vi "Set Subpanel Status.vi"(0 "GUI Container in":refnum<class "GUI Container.lvclass">, 5 "Subpanel":string, 9 "Subpanel Status":T1, 11 "error in (no error)":errorcluster) -> (4 "GUI Container out":refnum<class "GUI Container.lvclass">, 8 "Status Added":bool, 15 "error out":errorcluster)   [LabVIEW 2023, in "GUI Views.lvlib" / "GUI Container.lvclass"]
uses:
  GUI Container.lvclass
  typedefs/Subpanel Status.ctl
  GUI Container.lvclass/GUI Container.ctl
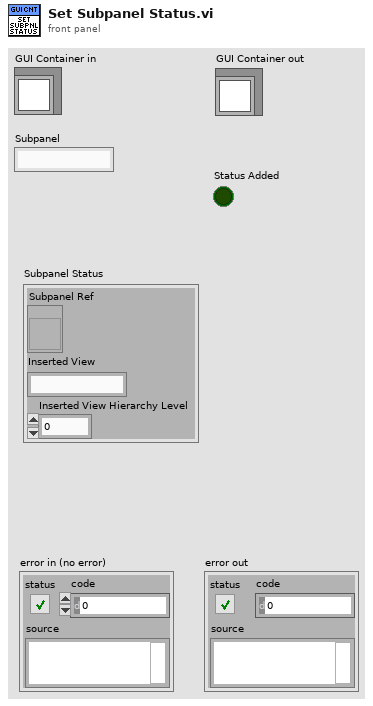
[diagram p1: front panel]
types:
  T1 = typedef "GUI Views.lvlib/GUI Container.lvclass/Subpanel Status.ctl" = cluster{"Subpanel Ref":refnum<vi>, "Inserted View":string, "Inserted View Hierarchy Level":i32}
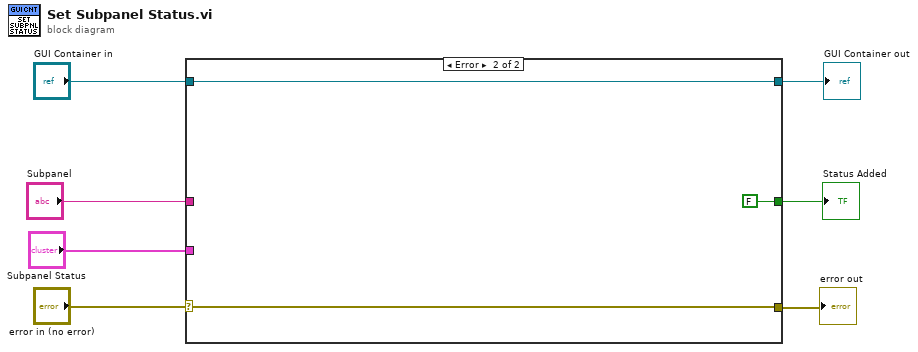
[diagram p0: block diagram]
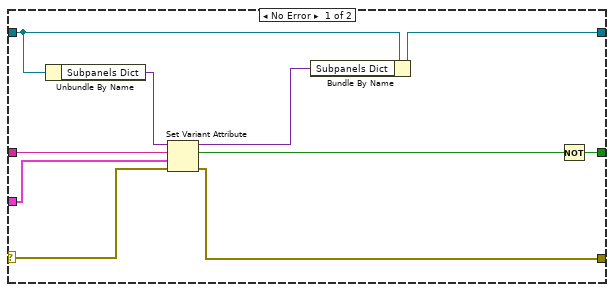
[diagram p2: hidden frame]
diagram:
  n1 = case shown="Error" "error in (no error)" {
    selector: "error in (no error)" -> [w15 w19]
    tunnel: [w13 w19] -> w7
    tunnel: "GUI Container in" -> [w16 w20]
    tunnel: "Subpanel" -> [w17 _]
    tunnel: [w11 w20] -> w3
    tunnel: [w8 FALSE] -> w2
    tunnel: "Subpanel Status" -> [w12 _]
    frame No Error {
      n2 = Unbundle By Name(w16) -> ("Subpanels Dict"=w14:variant)
      n3 = Set Variant Attribute(Variant=w14, name=w17, value=w12, error in=w15) -> (Variant out=w10:variant, replaced=w9:bool, error out=w13:errorcluster)
      n4 = Bundle By Name(cluster=w16, "Subpanels Dict"=w10) -> (w11:refnum<class "GUI Container.lvclass">)
      n5 = Not(x=w9) -> (.not. x?=w8:bool)
    }
    frame Error {
    }
  }
  "error out" <- w7
  "GUI Container out" <- w3
  "Status Added" <- w2
